vi "get_inputsFromLog.vi"(11 "String":string) -> (1 "joint=":string[](array[string]), 2 "input_camera":string[](array[string]), 3 "Array":string[](array[string]))   [LabVIEW 2022 SP3]
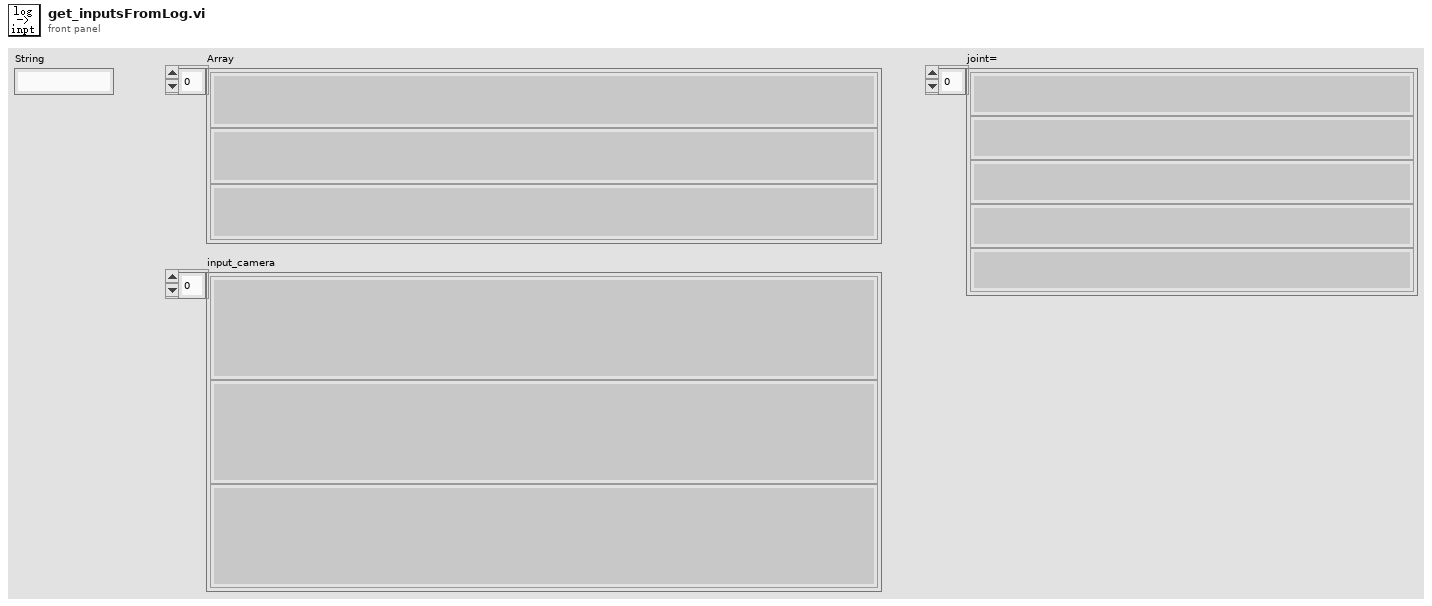
[diagram p1: front panel]
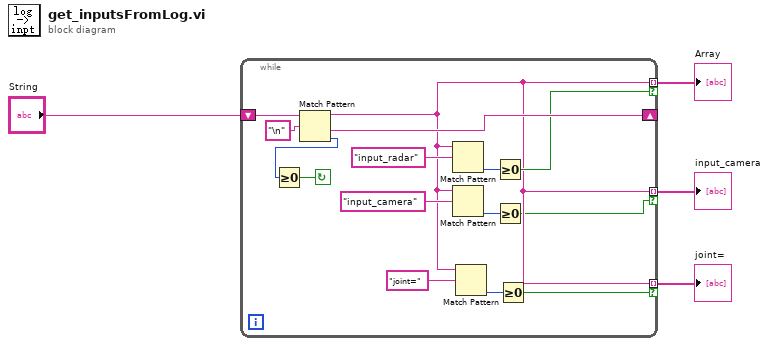
[diagram p0: block diagram]
diagram:
  n1 = while {
    shift-right: [w18] -> _
    shift-left: "String" -> [w19]
    tunnel: [w6] -> w3 mode=indexing if=w13
    tunnel: [w6] -> w1 mode=indexing if=w9
    tunnel: [w6] -> w2 mode=indexing if=w5
    stop <- w16 continue-if-true
    n2 = Match Pattern(string=w19, regular expression="\n") -> (before substring=w6:string, after substring=w18:string, offset past match=w15:i32)  [unwired: 1 in, 1 out]
    n3 = Greater Or Equal To 0?(x=w15) -> (x >= 0?=w16:bool)
    n4 = Match Pattern(string=w6, regular expression="input_radar") -> (offset past match=w14:i32)  [unwired: 1 in, 3 out]
    n5 = Match Pattern(string=w6, regular expression="input_camera") -> (offset past match=w7:i32)  [unwired: 1 in, 3 out]
    n6 = Match Pattern(string=w6, regular expression="joint=") -> (offset past match=w12:i32)  [unwired: 1 in, 3 out]
    n7 = Greater Or Equal To 0?(x=w14) -> (x >= 0?=w13:bool)
    n8 = Greater Or Equal To 0?(x=w7) -> (x >= 0?=w5:bool)
    n9 = Greater Or Equal To 0?(x=w12) -> (x >= 0?=w9:bool)
  }
  "Array" <- w3
  "input_camera" <- w2
  "joint=" <- w1
